vi "Write Current Position.vi"(8 "error in":errorcluster, 10 "Current Position":string, 11 "Gantry in":refnum<class "Gantry.lvclass">) -> (0 "error out":errorcluster, 3 "Gantry out":refnum<class "Gantry.lvclass">)   [LabVIEW 2024, in "Gantry.lvclass"]
uses:
  Gantry.lvclass
  Gantry.lvclass/Gantry.ctl
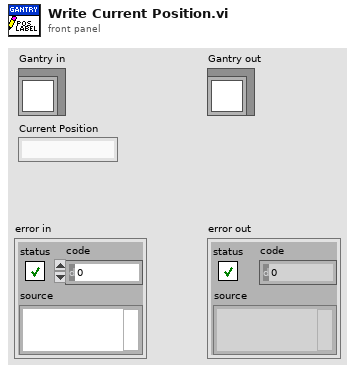
[diagram p1: front panel]
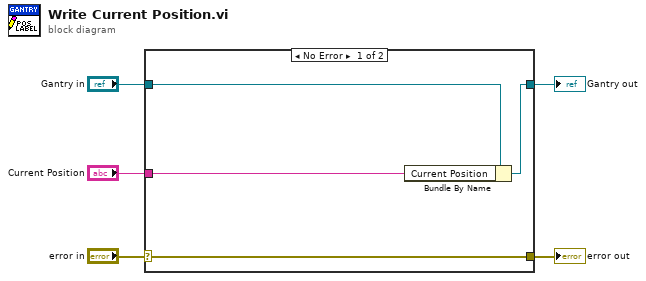
[diagram p0: block diagram]
diagram:
  n1 = case shown="No Error" "error in" {
    selector: "error in" -> [w9 w10]
    tunnel: [w9 w10] -> w4
    tunnel: [w7 w11] -> w2
    tunnel: "Gantry in" -> [w8 w11]
    tunnel: "Current Position" -> [w6 _]
    frame No Error {
      n2 = Bundle By Name(cluster=w8, "Current Position"=w6) -> (w7:refnum<class "Gantry.lvclass">)
    }
    frame Error {
    }
  }
  "error out" <- w4
  "Gantry out" <- w2
